vi "FT_Read_String_Data_64bit.vi"(4 "error in (no error)":errorcluster, 6 "Bytes To Read":u32, 7 "Handle":u64) -> (0 "error out":errorcluster, 1 "Bytes Read":u32, 2 "Read Data":string, 3 "Handle out":u64)   [LabVIEW 2019]
uses:
  FTD2XX.dll
panel:
  out "FT_Status":u32(ring) items=["FT_OK", "FT_INVALID_HANDLE", "FT_DEVICE_NOT_FOUND", "FT_DEVICE_NOT_OPENED", "FT_IO_ERROR", "FT_INSUFFICIENT_RESOURCES", "FT_INVALID_PARAMETER", "FT_INVALID_BAUD_RATE", "FT_DEVICE_NOT_OPENED_FOR_ERASE", "FT_DEVICE_NOT_OPENED_FOR_WRITE", "FT_FAILED_TO_WRITE_DEVICE", "FT_EEPROM_READ_FAILED", "FT_EEPROM_WRITE_FAILED", "FT_EEPROM_ERASE_FAILED", "FT_EEPROM_NOT_PRESENT", "FT_EEPROM_NOT_PROGRAMMED", "FT_INVALID_ARGS", "FT_NOT_SUPPORTED", "FT_OTHER_ERROR"]
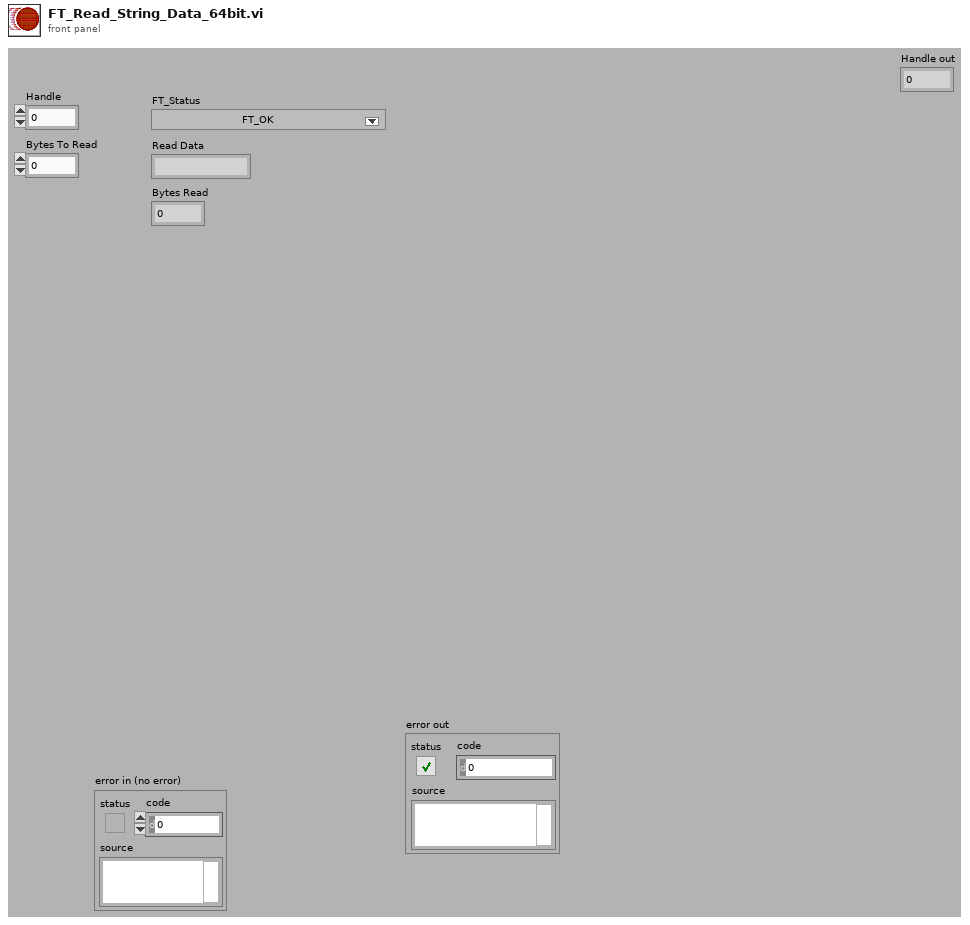
[diagram p1: front panel]
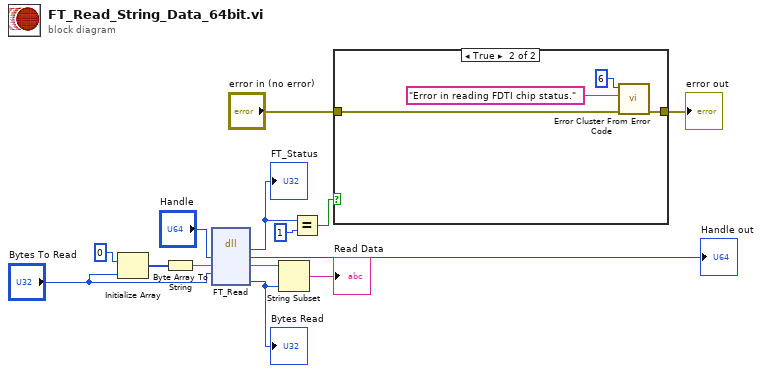
[diagram p0: block diagram]
diagram:
  n1 = Initialize Array(u8 0, "Bytes To Read") -> (w12:u8[])
  n2 = Byte Array To String(unsigned byte array=w12) -> (string=w11:string)
  n3 = dll-call lib="FTD2XX.dll" fn="FT_Read"("Handle"="Handle", "Buffer"=w11, "BytesToRead"="Bytes To Read") -> ("FT_Status"=w2:u32, "Handle"=→"Handle out":u64, "Buffer"=w8:string, "BytesReturned"=w7:u32)  [unwired: 5 in, 2 out]
  "FT_Status" <- w2
  "Bytes Read" <- w7
  n4 = String Subset(string=w8, length (rest)=w7) -> (substring=→"Read Data":string)  [unwired: 1 in]
  n5 = Equal?(x=w2, y=u32 1) -> (x = y?=w6:bool)
  n6 = case shown="True" w6 {
    tunnel: [w15 w18] -> w3
    tunnel: "error in (no error)" -> [w15 w17]
    frame False {
    }
    frame True {
      n7 = call <vilib>:"Error Cluster From Error Code.vi"("error in (no error)"=w17, "error message (\"\")"="Error in reading FDTI chip status." ("error message (\"\")"), "error code (0)"=6) -> ("error out"=w18:errorcluster)  [unwired: 6 in]
    }
  }
  "error out" <- w3
